vi "CLD 2  Elapsed Time Express with pause Solution.vi"() -> ()   [LabVIEW 2009]
doc: "Dieses VI veranschaulicht eine Möglichkeit, wie Funktionsumfang zum Pausieren der Zeitmessung zum Express-VI \"Verstrichene Zeit\" hinzugefügt werden kann. Bei dieser Methode wird der Eingang \"Startzeit festlegen\" verwendet, mit dessen Hilfe reelle Zeit gemessen und eine Pause eingefügt wird.\n\nEine andere Methode wäre z. B. das Messen der verstrichenen Zeit und Ändern der Zielzeit, wenn die Zeitmessung fortgesetzt wird. Diese Methode ist jedoch umständlich und führt zu zusätzlichem Overhead, wenn das VI die ursprüngliche Zielzeit anzeigen soll.\n\nBeschreibung der Ausführung der Case-Struktur \"'Änderung der Startzeit' anhalten\".\n\n\"FALSE\"-Case: Wird nicht angehalten, Standard-Timer\n\nDie aktuelle Zeit wird an das Schieberegister \"Kreislauf\" übergeben. Mit Hilfe der Zeit, die dem Ablauf wieder zugeführt wird, lässt sich feststellen, wann der Timer das letzte Mal noch nicht angehalten wurde. Außerdem wird damit die Zeitdifferenz am Ende der Pause ermittelt. Wird nicht verwendet, so lange die Schaltfläche \"Pause\" auf \"False\" gesetzt ist.\n\nDie \"Startzeit\" wird verwendet und weitergegeben. Sobald \"Zeit ist verstrichen\" TRUE ist, wird die neue aktuelle Zeit an die Startzeit übergeben.\n\n\"TRUE\"-Case: Pause-Schaltfläche ist gedrückt\nBerechnet die Zeitdifferenz zwischen dem letzten Mal, als die Pause-Schaltfläche \"FALSE\" war (Kreislaufzeit) und der aktuellen Zeit. Addiert die Zeitdifferenz (Verweildauer während der Pause) zur Startzeit des Timers, d. h. die Startzeit verstreicht.\n\nDas Schieberegister \"Kreislaufzeit\" enthält immer noch den Wert für die aktuelle Zeit."
panel:
  out "Verstrichene Zeit (s)":dbl format="%#.1g"
  out "Zeit ist verstrichen":bool
  in  "Autom. zurücksetzen":bool
  in  "Pause-Schaltfläche":bool
  in  "Zurücksetzen-Schaltfläche":bool
  in  "VI anhalten":bool
  out "Fehler (Ausgang)":errorcluster
  in  "Fehler (Eingang)":errorcluster
  in  "Zielzeit (s)":dbl
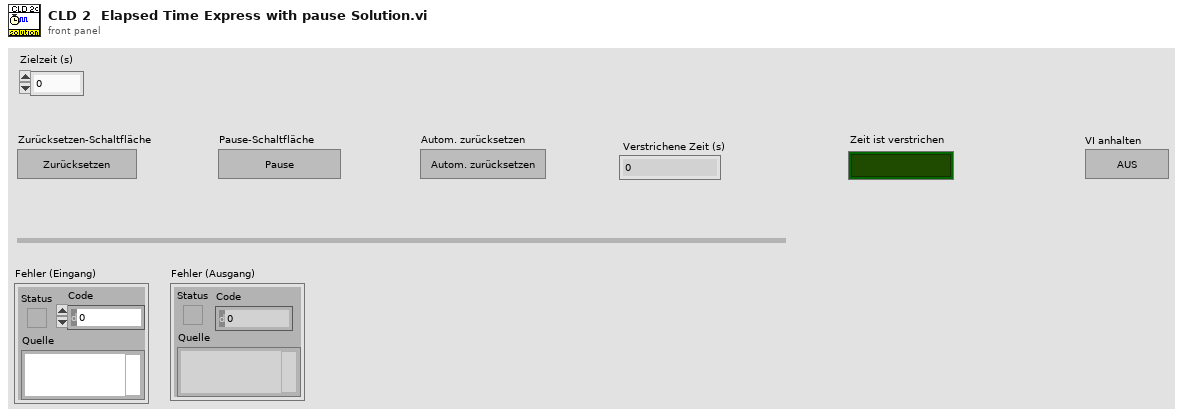
[diagram p1: front panel]
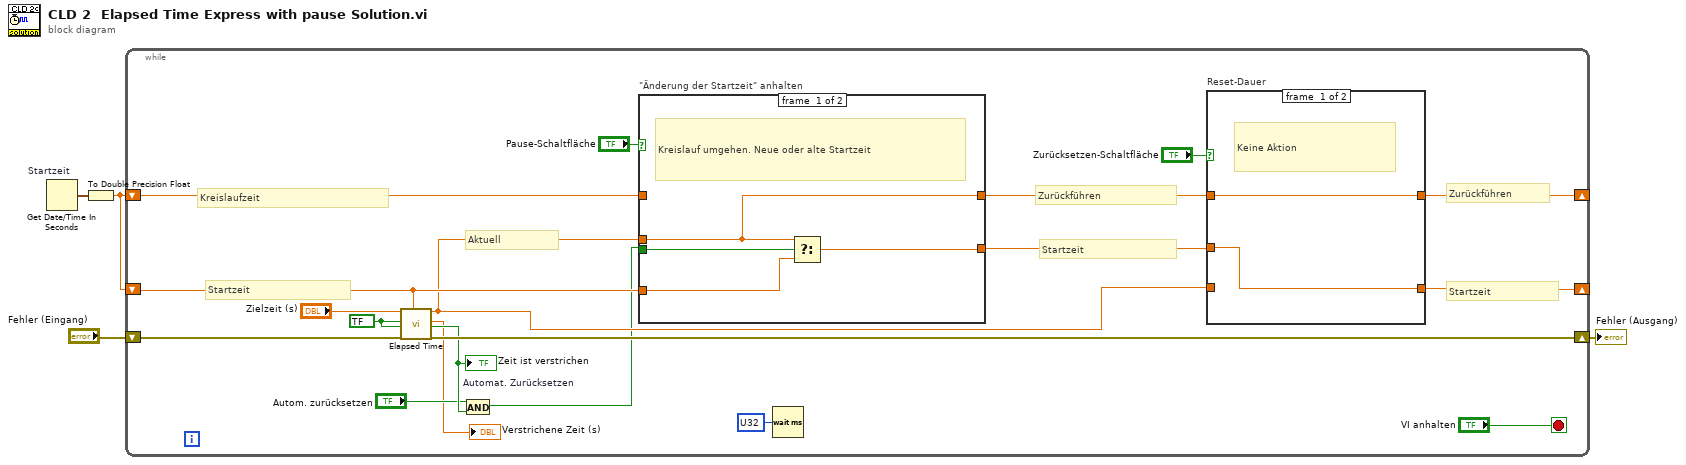
[diagram p0: block diagram]
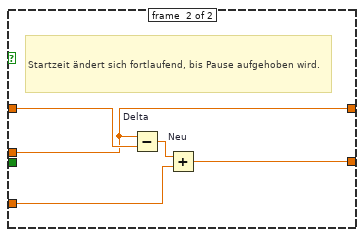
[diagram p3: hidden frame]
diagram:
  n1 = Get Date/Time In Seconds "Startzeit"() -> (seconds since 1Jan1904=w2:timestamp)
  n2 = To Double Precision Float(number=w2) -> (double precision float=w1:dbl)
  n3 = while {
    shift-right: [w11] -> _
    shift-left: w1 -> [w20]
    shift-right: [w17] -> w3
    shift-left: "Fehler (Eingang)" -> [w18]
    shift-right: [w13] -> _
    shift-left: w1 -> [w16]
    stop <- "VI anhalten" stop-if-true
    w8 = bool ? ("Zurücksetzen")
    # "Aktuell"
    # "Startzeit"
    # "Kreislaufzeit"
    # "Zurückführen"
    # "Zurückführen"
    # "Startzeit"
    # "Startzeit"
    n4 = call "Elapsed Time"("Time Target (s)"="Zielzeit (s)", "Reset"=w8, "Auto Reset"=w8, "error in (no error)"=w18, "Set Start Time (s)"=w20) -> ("Present (s)"=w10:dbl, "Elapsed Time (s)"=→"Verstrichene Zeit (s)":dbl, "Time has Elapsed"=w9:bool, "error out"=w17:errorcluster)  [unwired: 7 in, 4 out]
    "Zeit ist verstrichen" <- w9
    n5 = And "Automat. Zurücksetzen"(x="Autom. zurücksetzen", y=w9) -> (x .and. y?=w7:bool)
    n6 = case "\"Änderung der Startzeit\" anhalten" shown="True" "Pause-Schaltfläche" {
      tunnel: w7 -> [w30 _]
      tunnel: w10 -> [w27 w31]
      tunnel: [w29 w33] -> w12
      tunnel: w20 -> [w28 w32]
      tunnel: [w27 w31] -> w14
      tunnel: w16 -> [_ w34]
      frame #0 {
        # "Kreislauf umgehen. Neue oder alte Startzeit"
        n7 = Select(t=w27, s=w30, f=w28) -> (s? t:f=w29:dbl)
      }
      frame #1 {
        # "Startzeit ändert sich fortlaufend, bis Pause aufgehoben wird."
        n8 = Subtract "Delta"(x=w31, y=w34) -> (x-y=w35:dbl)
        n9 = Add "Neu"(x=w35, y=w32) -> (x+y=w33:dbl)
      }
    }
    n10 = Wait (ms)(milliseconds to wait=u32 ? ("Zu wartende ms")) -> ()  [unwired: 1 out]
    n11 = case "Reset-Dauer" shown="True" "Zurücksetzen-Schaltfläche" {
      tunnel: [w25 w26] -> w13
      tunnel: w14 -> [w25 _]
      tunnel: [w24 w26] -> w11
      tunnel: w12 -> [w24 _]
      tunnel: w10 -> [_ w26]
      frame #0 {
        # "Keine Aktion"
      }
      frame #1 {
        # "Beide Zeiten werden auf den gleichen Wert gesetzt"
      }
    }
  }
  "Fehler (Ausgang)" <- w3
